vi "Set SG Path.vi"(0 "Path in":refnum<class "SG 8GHz Path.lvclass">, 5 "Cal point in":T1, 11 "error in":errorcluster) -> (4 "Path out":refnum<class "SG 8GHz Path.lvclass">, 6 "Cal point out":T1, 8 "Source Gain":dbl, 10 "Digital Gain":dbl, 15 "error out":errorcluster)   [LabVIEW 2023, in "RFFixtureCharact.RMM.lvlib" / "SG 8GHz Path.lvclass"]
uses:
  SG 8GHz Path.lvclass
  Public/Base Classes/Scalar/Scalar Path/Type Definitions/Cal Point.ctl
  SG 8GHz Path.lvclass/SG 8GHz Path.ctl
  Public/Base Classes/Scalar/SG Path/SG Path.lvclass
  Public/Base Classes/Scalar/Scalar Path/Scalar Path.lvclass
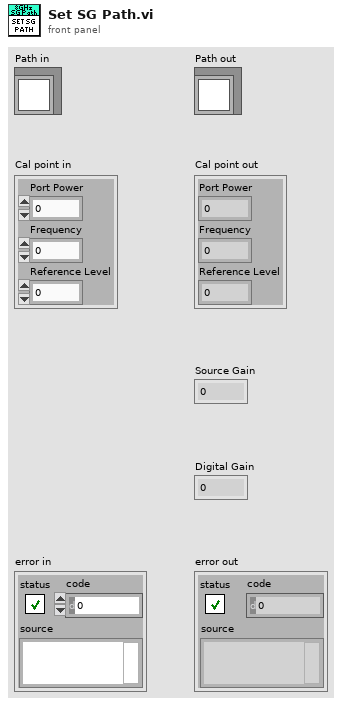
[diagram p1: front panel]
types:
  T1 = typedef "RFFixtureCharact.Public.lvlib/Scalar Path.lvclass/Cal Point.ctl" = cluster{"Port Power":dbl, "Frequency":dbl, "Reference Level":dbl}
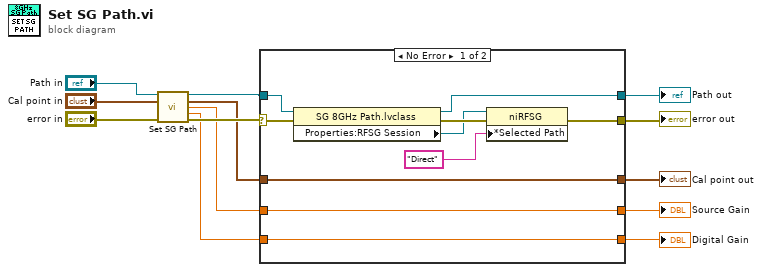
[diagram p0: block diagram]
diagram:
  n1 = call-parent "Set SG Path.vi"("Path in"="Path in", "Cal point in"="Cal point in", "error in"="error in") -> ("Path out"=w8:refnum<class "SG 8GHz Path.lvclass">, "Cal point out"=w6:T1, "Source Gain"=w5:dbl, "Digital Gain"=w4:dbl, "error out"=w10:errorcluster)  [unwired: 8 in]
  n2 = case shown="No Error" w10 {
    selector: w10 -> [w23 w28]
    tunnel: w8 -> [w22 w27]
    tunnel: [w19 w27] -> w7
    tunnel: [w18 w28] -> w9
    tunnel: [w16 w26] -> w3
    tunnel: w6 -> [w16 w26]
    tunnel: [w15 w25] -> w1
    tunnel: w5 -> [w15 w25]
    tunnel: [w14 w24] -> w2
    tunnel: w4 -> [w14 w24]
    frame No Error {
      n3 = property class="SG 8GHz Path.lvclass"(reference=w22, error in=w23) -> (reference out=w19:refnum<class "SG 8GHz Path.lvclass">, error out=w21:errorcluster, "Properties:RFSG Session"=w20:refnum<k15>)
      n4 = property class="niRFSG"(reference=w20, error in=w21, "*Selected Path"="Direct" ("Private:Device Specific:Vector Signal Transceiver:Signal Path:Selected Path")) -> (error out=w18:errorcluster)  [unwired: 1 out]
    }
    frame Error {
    }
  }
  "error out" <- w9
  "Source Gain" <- w1
  "Cal point out" <- w3
  "Digital Gain" <- w2
  "Path out" <- w7
